vi "FGV_SimpleNumericWithAE.vi"(10 "Numeric":i32, 11 "Mode":enum16{"SET", "GET", "INCREMENT", "DECREMENT"}(ring)) -> (2 "Numeric Out":i32)   [LabVIEW 2020]
doc: "Example of GET/SET Functional Global Variabl with numeric data. This FGBV contains action engine with decrement and increment function. Comments in Polish."
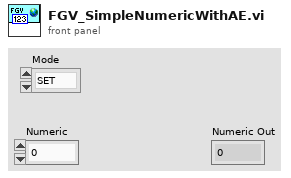
[diagram p1: front panel]
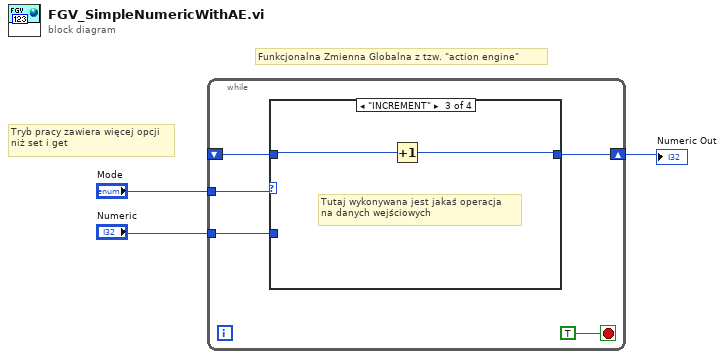
[diagram p0: block diagram]
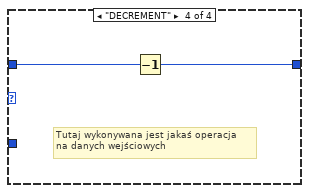
[diagram p4: hidden frame]
diagram:
  # "Tryb pracy zawiera więcej opcji\nniż set i get"
  # "Funkcjonalna Zmienna Globalna z tzw. \"action engine\""
  n1 = while {
    tunnel: "Mode" -> [w7]
    shift-right: [w5] -> w1
    shift-left: _ -> [w4]
    tunnel: "Numeric" -> [w6]
    stop <- TRUE stop-if-true
    n2 = case shown="\"INCREMENT\"" w7 {
      tunnel: w6 -> [w9 _ _ _]
      tunnel: [w9 w10 w11 w13] -> w5
      tunnel: w4 -> [_ w10 w12 w14]
      frame "SET", Default {
      }
      frame "GET" {
      }
      frame "INCREMENT" {
        # "Tutaj wykonywana jest jakaś operacja \nna danych wejściowych"
        n3 = Increment(x=w12) -> (x+1=w11:i32)
      }
      frame "DECREMENT" {
        # "Tutaj wykonywana jest jakaś operacja \nna danych wejściowych"
        n4 = Decrement(x=w14) -> (x-1=w13:i32)
      }
    }
  }
  "Numeric Out" <- w1
